vi "WorkingSimpleExample.vi"() -> ()   [LabVIEW 2020]
uses:
  C887 DLL/Low Level/Communication.llb/Interface Settings.ctl
panel:
  out "Velocity":dbl[](array[numeric]) format="%.6f"
  in  "Velocity":bool
  out "Was connected?":bool
  in  "Close Connection":bool
  out "Move possible":bool
  out "Axis moving?":bool[](array[boolean])
  in  "Pivot point coordinates 2":cluster{"R":dbl, "S":dbl, "T":dbl} {"T" format="%.4f"; "S" format="%.4f"; "R" format="%.4f"}
  out "Pivot point coordinates":cluster{"R":dbl, "S":dbl, "T":dbl} {"T" format="%.4f"; "S" format="%.4f"; "R" format="%.4f"}
  in  "Pivot":bool
  out "Axis status":dbl[](array[numeric])
  in  "Status":bool
  in  "Zero Position":bool
  out "Target position":dbl[](array[numeric]) format="%.6f"
  in  "Axes to move":string[](array[string])
  in  "Position values":dbl[](array[numeric]) format="%.6f"
  in  "Move Position":bool
  out "Position":dbl[](array[numeric]) format="%.6f"
  in  "Read Position":bool
  in  "Initialize":bool
  in  "stop":bool
  out "Conn. Axes out":string[](array[string])
  in  "Interface settings":T1={"Interface"=0, "Timeout"=5000, "RS232 settings"={"Portnumber"=1, "Baudrate"=5}, "TCP/IP settings"={"Host address/name"="localhost", "Port"=50000, "Board"=0, "TCP/IP Search?"=TRUE}, "USB settings"={"S/N"="", "USB Search?"=TRUE}, "DaisyChain settings"={"Register DC"=FALSE, "DaisyChain Search?"=TRUE, "Device ID"=1}, "DLL for Device"=0} {"DLL for Device" items=["None", "C-843", "C-844", "E-710", "C-843.PM", "C-865", "E-761", "Mercury", "E-755", "E-753", "C-866", "E-712", "E-725", "E-861", "C-867", "E-517", "E-816", "E-709", "PI_GCS2_DLL", "HydraPollux"]; "Interface" items=["RS232", "RS232 DaisyChain", "USB", "USB DaisyChain", "TCP/IP", "TCP/IP DaisyChain", "PCI"]; "RS232 settings"."Portnumber" min=1 step=1; "RS232 settings"."Baudrate" items=["9600", "14400", "19200", "38400", "57600", "115200", "230400", "460800"]}
  out "error in 2":errorcluster
  in  "error in":errorcluster
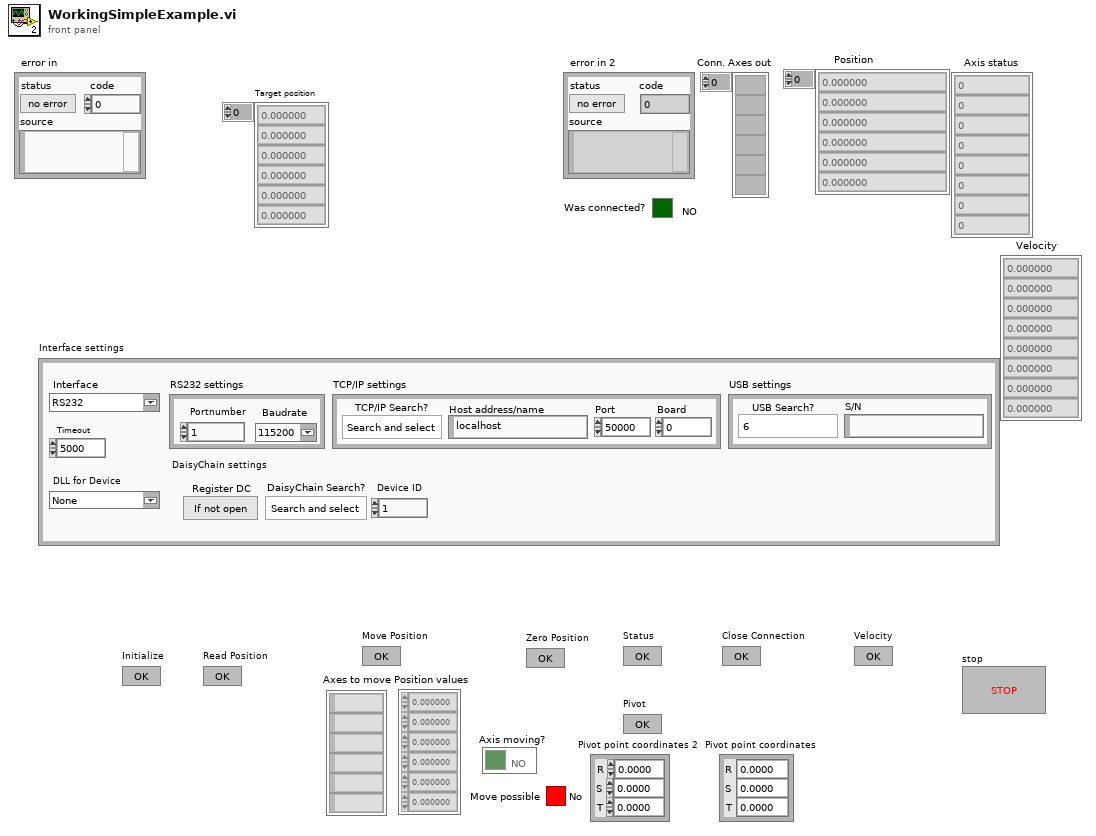
[diagram p1: front panel]
types:
  T1 = typedef "Interface Settings.ctl" = cluster{"Interface":u16, "Timeout":u32, "RS232 settings":cluster{"Portnumber":u8, "Baudrate":u16}, "TCP/IP settings":cluster{"Host address/name":string, "Port":i32, "Board":i32, "TCP/IP Search?":bool}, "USB settings":cluster{"S/N":string, "USB Search?":bool}, "DaisyChain settings":cluster{"Register DC":bool, "DaisyChain Search?":bool, "Device ID":i32}, "DLL for Device":u16}
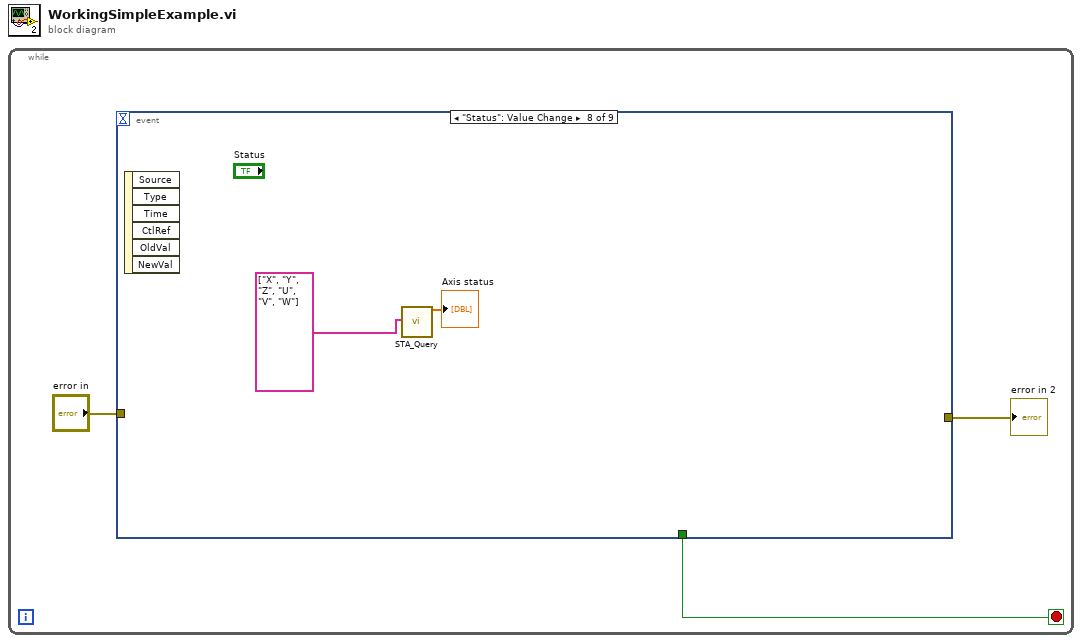
[diagram p0: block diagram]
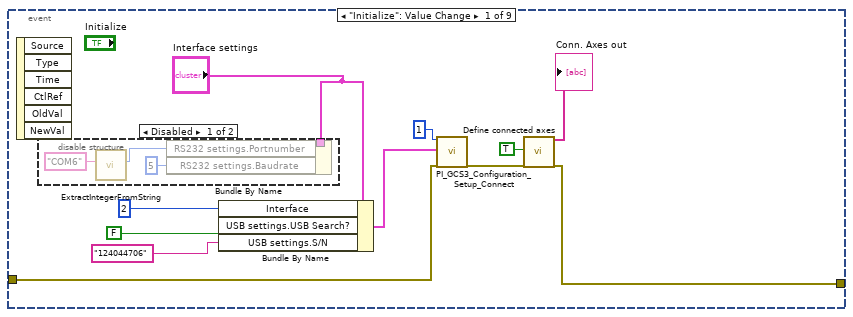
[diagram p2: hidden frame]
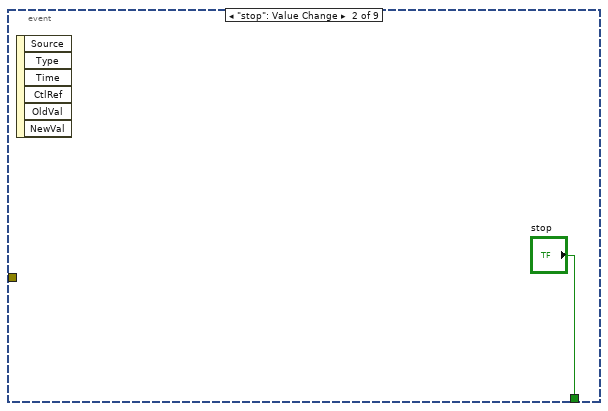
[diagram p4: hidden frame]
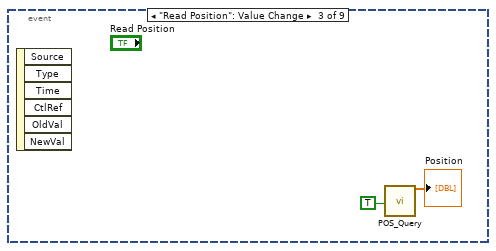
[diagram p5: hidden frame]
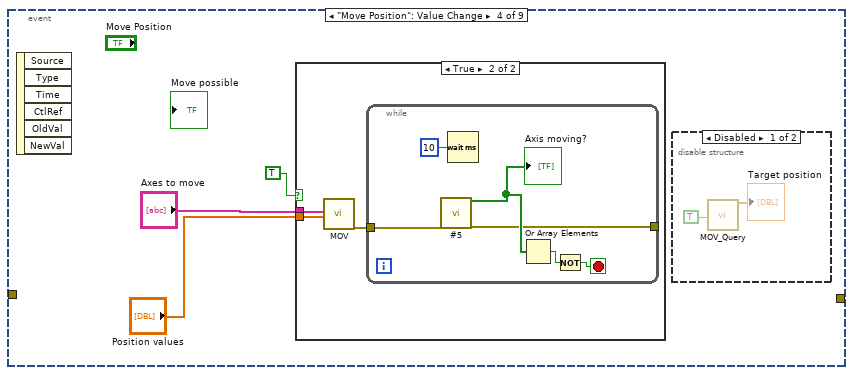
[diagram p6: hidden frame]
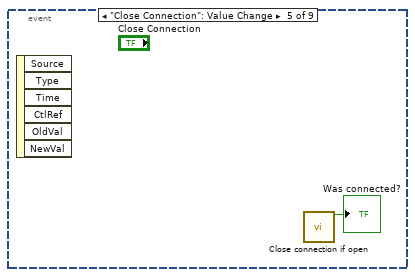
[diagram p9: hidden frame]
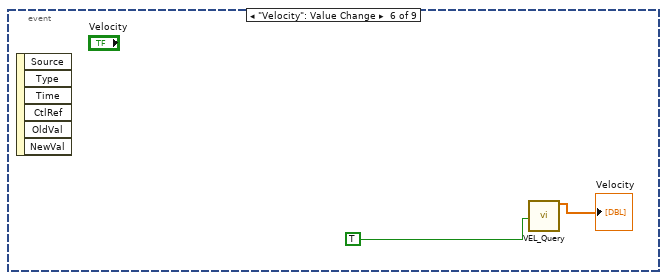
[diagram p10: hidden frame]
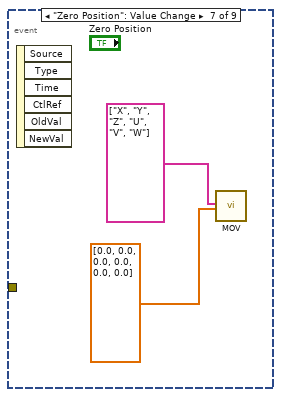
[diagram p11: hidden frame]
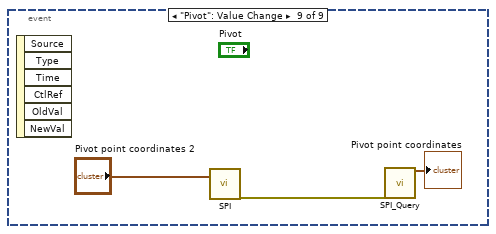
[diagram p12: hidden frame]
diagram:
  n1 = while {
    stop <- w1 stop-if-true
    n2 = event shown="[7] \"Status\": Value Change" {
      selector: _ -> [_ _ _ _ _ _ _ _ _]
      dyn-events: _ -> [_ _ _ _ _ _ _ _ _]
      timeout: _ -> [_ _ _ _ _ _ _ _ _]
      tunnel: [w10 _ _ _ _ _ _ _ _] -> w3
      tunnel: "error in" -> [w9 _ _ _ _ _ _ _ _]
      tunnel: [_ "stop" _ _ _ _ _ _ _] -> w1
      event "Initialize": Value Change {
        n3 = event-data() -> ()  [unwired: 1 in, 6 out]
        n4 = disable-structure shown="Disabled" {
          disable-tunnel: "Interface settings" -> [w15 _]
          frame Disabled {
            n5 = call "ExtractIntegerFromString.vi"("String"="COM6") -> ("number"=w17:i32)  [unwired: 10 in]
            n6 = Bundle By Name(cluster=w15, "RS232 settings.Portnumber"=w17, "RS232 settings.Baudrate"=u16 5) -> ()  [unwired: 1 out]
          }
          frame Enabled {
          }
        }
        n7 = Bundle By Name(cluster="Interface settings", "Interface"=u16 2, "USB settings.USB Search?"=FALSE, "USB settings.S/N"="124044706") -> (w7:T1)
        n8 = call "PI_GCS3_Configuration_Setup_Connect.vi"("System no."=1, "Interface settings"=w7, "error in"=w9) -> ("error out"=w13:errorcluster)  [unwired: 16 in]
        n9 = call "Define connected axes.vi"("Read from\ncontroller?"=TRUE ("Read from\ncontroller?"), "error in"=w13) -> ("Conn. Axes out"=→"Conn. Axes out":string[], "error out"=w10:errorcluster)  [unwired: 16 in]
      }
      event "stop": Value Change {
        n10 = event-data() -> ()  [unwired: 1 in, 6 out]
      }
      event "Read Position": Value Change {
        n11 = event-data() -> ()  [unwired: 1 in, 6 out]
        n12 = call "POS_Query.vi"("All axes?"=TRUE) -> ("Position"=→"Position":dbl[])  [unwired: 17 in, 1 out]
      }
      event "Move Position": Value Change {
        n13 = event-data() -> ()  [unwired: 1 in, 6 out]
        n14 = case shown="True" TRUE {
          tunnel: "Axes to move" -> [_ w29]
          tunnel: "Position values" -> [_ w28]
          frame False {
          }
          frame True {
            n15 = call "MOV.vi"("Axes to move"=w29, "Position values"=w28) -> ("error out"=w27:errorcluster)  [unwired: 17 in]
            n16 = while {
              tunnel: w27 -> [w31]
              tunnel: [w30] -> _
              stop <- w32 stop-if-true
              n17 = call "#5.vi"("error in"=w31) -> ("Axis moving?"=w34:bool[], "error out"=w30:errorcluster)  [unwired: 17 in]
              "Axis moving?" <- w34
              n18 = Wait (ms)(milliseconds to wait=u32 10) -> ()  [unwired: 1 out]
              n19 = Or Array Elements(Boolean array=w34) -> (logical OR=w33:bool)
              n20 = Not(x=w33) -> (.not. x?=w32:bool)
            }
          }
        }
        n21 = disable-structure shown="Disabled" {
          frame Disabled {
            n22 = call "MOV_Query.vi"("All axes?"=TRUE) -> ("Target position"=→"Target position":dbl[])  [unwired: 17 in, 1 out]
          }
          frame Enabled {
          }
        }
      }
      event "Close Connection": Value Change {
        n23 = event-data() -> ()  [unwired: 1 in, 6 out]
        n24 = call "Close connection if open.vi"() -> ("Was connected?"=→"Was connected?":bool)  [unwired: 18 in, 1 out]
      }
      event "Velocity": Value Change {
        n25 = event-data() -> ()  [unwired: 1 in, 6 out]
        n26 = call "VEL_Query.vi"("All axes?"=TRUE) -> ("Velocity"=→"Velocity":dbl[])  [unwired: 17 in, 1 out]
      }
      event "Zero Position": Value Change {
        n27 = event-data() -> ()  [unwired: 1 in, 6 out]
        n28 = call "MOV.vi"("Axes to move"=string[] ["X", "Y", "Z", "U", "V", "W"], "Position values"=dbl[] [0.0, 0.0, 0.0, 0.0, 0.0, 0.0]) -> ()  [unwired: 17 in, 1 out]
      }
      event "Status": Value Change {
        n29 = event-data() -> ()  [unwired: 1 in, 6 out]
        n30 = call "STA_Query.vi"("Axes to query"=string[] ["X", "Y", "Z", "U", "V", "W"] ("Axes to move")) -> ("Axis status"=→"Axis status":dbl[])  [unwired: 17 in, 1 out]
      }
      event "Pivot": Value Change {
        n31 = event-data() -> ()  [unwired: 1 in, 6 out]
        n32 = call "SPI.vi"("Pivot point coordinates"="Pivot point coordinates 2") -> ("error out"=w43:errorcluster)  [unwired: 17 in, 1 out]
        n33 = call "SPI_Query.vi"("error in"=w43) -> ("Pivot point coordinates"=→"Pivot point coordinates":cluster{"R":dbl, "S":dbl, "T":dbl})  [unwired: 17 in, 1 out]
      }
    }
    "error in 2" <- w3
  }
